vi "Add.vi"() -> ()   [LabVIEW 2016]
panel:
  out "C":dbl
  in  "B":dbl=5.0
  in  "A":dbl=2.0
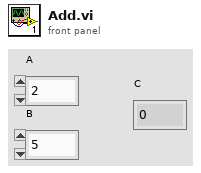
[diagram p1: front panel]
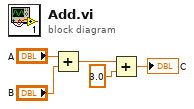
[diagram p0: block diagram]
diagram:
  n1 = Add(x="A", y="B") -> (x+y=w3:dbl)
  n2 = Add(x=w3, y=3.0) -> (x+y=→"C":dbl)
